vi "Init_Test.vi"(8 "error in (no error)":errorcluster caption="entrée d'erreur (pas d'erreur)", 11 "Print_Label en entrée":refnum<class "Close_Instr.lvclass">) -> (0 "error out":errorcluster caption="sortie d'erreur", 3 "Print_Label en sortie":refnum<class "Close_Instr.lvclass">)   [LabVIEW 2020, in "Library Test.lvlib" / "Close_Instr.lvclass"]
uses:
  Close_Instr.lvclass
  C:/Users/ngarcin/OneDrive - Altyor/Standard TB/Class/Test/Test (Default)/Test (Default).lvclass
  Commun VI/TypeDef/Commande Test/Commande Value Type.ctl
  Commun VI/TypeDef/Commande Test/Commande Type Test.ctl
  Test_Wtih_Instr/Test_With_Inst.lvclass
  Instrument/Instrument (Default)/Class Instrument (Default).lvclass
  Close_Instr.lvclass/Close_Instr.ctl
  Commun VI/Library Commun.lvlib
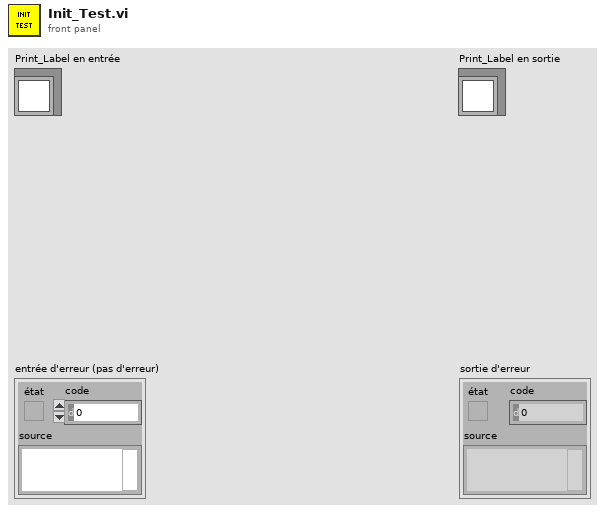
[diagram p1: front panel]
types:
  T1 = typedef "Library Commun.lvlib/Commande Type Test.ctl" = enum16{"Function", "Test", "Calculation"}
  T2 = typedef "Library Commun.lvlib/Commande Value Type.ctl" = enum16{"None", "String", "Number", "Timestamp", "Boolean", "Array"}
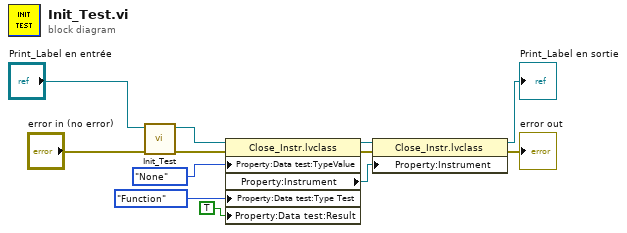
[diagram p0: block diagram]
diagram:
  n1 = call-parent "Init_Test.vi"("error in (no error)"="error in (no error)", "Test_With_Inst en entrée"="Print_Label en entrée") -> ("error out"=w9:errorcluster, "Test_With_Inst en sortie"=w10:refnum<class "Close_Instr.lvclass">)  [unwired: 8 in]
  n2 = property class="Close_Instr.lvclass"(reference=w10, error in=w9, "Property:Data test:TypeValue"=Commande_Value_Type."None" ("TypeValue"), "Property:Data test:Type Test"=Commande_Type_Test."Function" ("Type Test"), "Property:Data test:Result"=TRUE ("Result")) -> (reference out=w8:refnum<class "Close_Instr.lvclass">, error out=w1:errorcluster, "Property:Instrument"=w2:refnum<class "Class Instrument (Default).lvclass">)
  n3 = property class="Close_Instr.lvclass"(reference=w8, error in=w1, "Property:Instrument"=w2) -> (reference out=→"Print_Label en sortie":refnum<class "Close_Instr.lvclass">, error out=→"error out":errorcluster)
